vi "SimulateButtonPress.vi"(8 "error in (no error)":errorcluster, 10 "VIRef":refnum<vi>, 11 "BooleanCtrlRef":refnum<vi>) -> (0 "error out":errorcluster)   [LabVIEW 2016]
panel:
  in  "Right-click?":bool
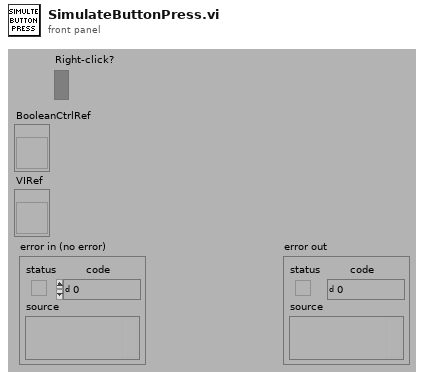
[diagram p1: front panel]
types:
  T1 = typedef "LVPositionTypeDef.ctl" = cluster{"Left":i32, "Top":i32}
  T2 = typedef "LVBoundsTypeDef.ctl" = cluster{"Width":u32, "Height":u32}
  T3 = typedef "LVRectTypeDef.ctl" = cluster{"Left":i16, "Top":i16, "Right":i16, "Bottom":i16}
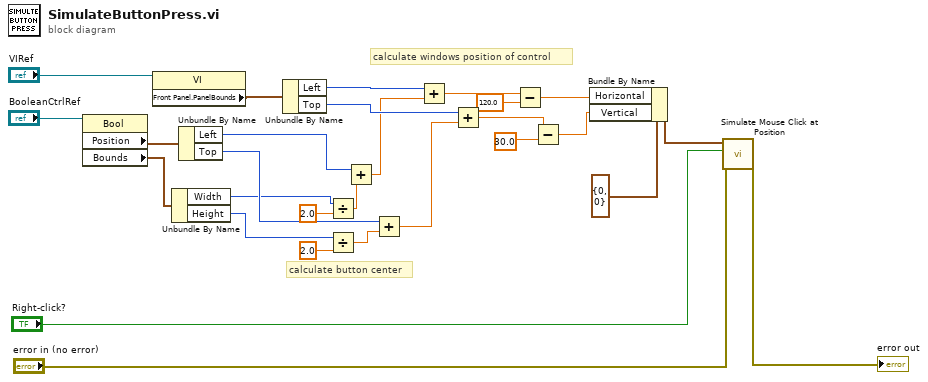
[diagram p0: block diagram]
diagram:
  # "calculate windows position of control"
  # "calculate button center"
  n1 = property on="Property Node" class="Bool"(reference="BooleanCtrlRef") -> ("Position"=w26:T1, "Bounds"=w20:T2)  [unwired: 1 in, 2 out]
  n2 = property class="VI"(reference="VIRef") -> ("Front Panel.PanelBounds"=w27:T3)  [unwired: 1 in, 2 out]
  n3 = Unbundle By Name(w20) -> ("Width"=w17:u32, "Height"=w11:u32)
  n4 = Unbundle By Name(w26) -> ("Left"=w16:i32, "Top"=w18:i32)
  n5 = Unbundle By Name(w27) -> ("Left"=w25:i16, "Top"=w24:i16)
  n6 = Divide(x=w17, y=2.0) -> (x/y=w15:dbl)
  n7 = Divide(x=w11, y=2.0) -> (x/y=w13:dbl)
  n8 = Add(x=w16, y=w15) -> (x+y=w14:dbl)
  n9 = Add(x=w18, y=w13) -> (x+y=w12:dbl)
  n10 = Add(x=w25, y=w14) -> (x+y=w6:dbl)
  n11 = Add(x=w24, y=w12) -> (x+y=w4:dbl)
  n12 = Subtract(x=w6, y=120.0) -> (x-y=w5:dbl)
  n13 = Subtract(x=w4, y=30.0) -> (x-y=w2:dbl)
  n14 = Bundle By Name(cluster=cluster{"Horizontal":i32, "Vertical":i32} {"Horizontal"=0, "Vertical"=0} ("Mouse Position"), "Horizontal"=w5, "Vertical"=w2) -> (w23:cluster{"Horizontal":i32, "Vertical":i32})
  n15 = call "Simulate Mouse Click at Position .vi"("error in (no error)"="error in (no error)", "Right-click?"="Right-click?", "Mouse Position"=w23) -> ("error out"=→"error out":errorcluster)  [unwired: 8 in]
